vi "Tower Immediate.vi"(7 "Description":string, 8 "Command Info In":T1, 9 "Deadband Value":dbl=0.01, 11 "Setpoint":dbl) -> (0 "Command Info Out":T1)   [LabVIEW 2017]
doc: "This template includes code for deadband comparision to avoid excessive command scheduling. It is particularly useful for joystick-driven commands.\n\nBe sure to right-click and select New from Template and save with a new command name."
uses:
  <vilib>/Rock Robotics/WPI/Framework/Command Status Info.ctl
  <vilib>/Rock Robotics/WPI/Framework/Completion Status.ctl
  <vilib>/Rock Robotics/WPI/Framework/Completion Notifier.ctl
  Implementation/tower Setpoints.ctl
  Implementation/tower Operations.ctl
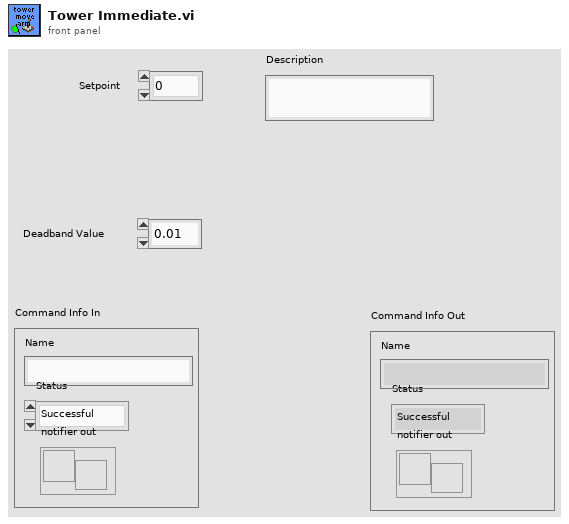
[diagram p1: front panel]
types:
  T1 = typedef "Command Status Info.ctl" = cluster{"Name":string, "Status":T2, "notifier out":T3}
  T2 = typedef "Completion Status.ctl" = enum16{"Successful", "Aborted", "Incomplete"}
  T3 = typedef "Completion Notifier.ctl" = refnum<notifier>
  T4 = typedef "tower Setpoints.ctl" = cluster{"Operation":T5, "Setpoint":dbl, "Duration":dbl}
  T5 = typedef "tower Operations.ctl" = enum16{"Reserve", "Read Current", "Immediate", "LaunchClimber", "ArmReset", "ArmPosition", "TowerClimbImmediate"}
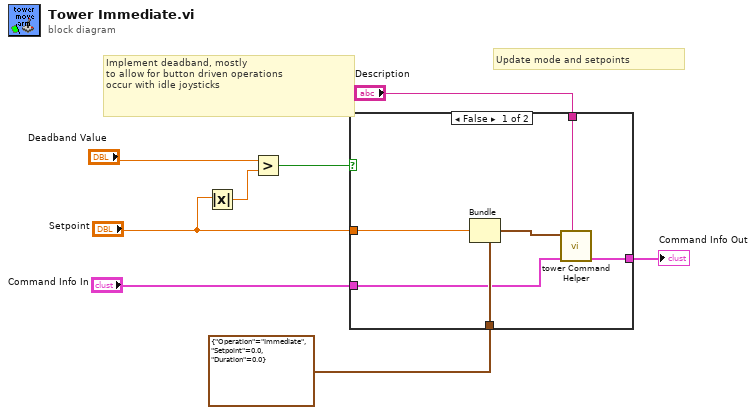
[diagram p0: block diagram]
diagram:
  # "Implement deadband, mostly\nto allow for button driven operations\noccur with idle joysticks"
  # "Update mode and setpoints"
  n1 = Absolute Value(x="Setpoint") -> (abs(x)=w7:dbl)
  n2 = Greater?(x="Deadband Value", y=w7) -> (0:w1:bool)
  n3 = case shown="False" w1 {
    tunnel: "Setpoint" -> [w14 _]
    tunnel: T4 {"Operation"=enum."Immediate", "Setpoint"=0.0, "Duration"=0.0} ("SubSystem Data") -> [w13 _]
    tunnel: [w12 w15] -> w6
    tunnel: "Command Info In" -> [w11 w15]
    tunnel: "Description" -> [w9 _]
    frame False {
      n4 = Bundle(cluster=w13, "Setpoint"=w14) -> (w10:T4)  [unwired: 2 in]
      n5 = call "tower Command Helper.vi"("Description"=w9, "Command Info In"=w11, "SubSystem Data"=w10) -> ("Command Info Out"=w12:T1)  [unwired: 6 in, 2 out]
    }
    frame True {
    }
  }
  "Command Info Out" <- w6
